vi "ObserverPattern_Demo_Main.vi"() -> ()   [LabVIEW 2010]
uses:
  WeatherData.ctl
  ForecastConditionDisplay_class/ForecastConditionDisplay.lvclass
  CurrentConditionDisplay_class/CurrentConditionDisplay.lvclass
  WeatherStation_class/WeatherStation.lvclass
panel:
  out "No.OfObservers":i32
  in  "Forecast.Subscribe?":bool caption="Subscribe?"
  in  "Subscribe?":bool
  out "Forecast message":string
  out "Forecast Temperature F":dbl(slide) scale=0.0..160.0
  out "Forecast":string
  out "Humid %":dbl(knob) scale=0.0..100.0
  out "CurrentTemperature C":dbl(slide) scale=0.0..60.0
  in  "stop":bool
  in  "error in (no error)":errorcluster
  in  "WeatherData-Acquired":T1
  # "CURRENT CONDITION"
  # "FORECAST"
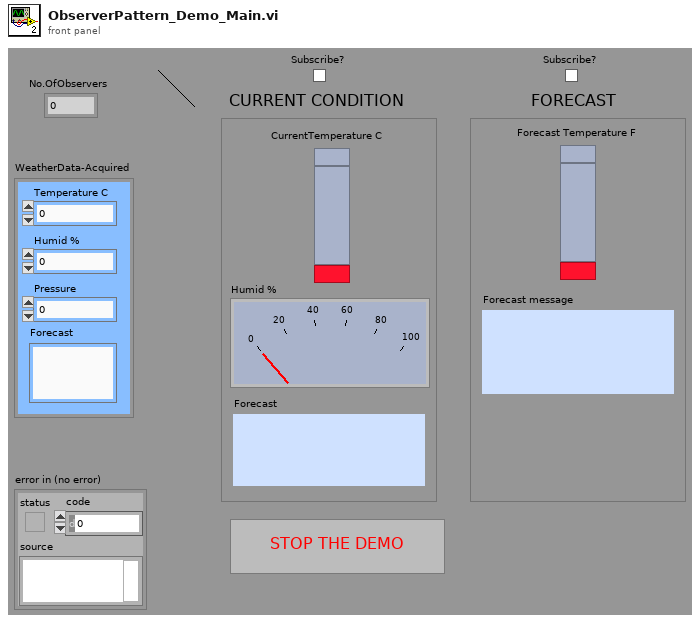
[diagram p1: front panel]
types:
  T1 = typedef "WeatherData.ctl" = cluster{"Temperature C":dbl, "Humid %":dbl, "Pressure":dbl, "Forecast":string}
  T2 = cluster{"No.OfObservers":i32, "CurrentDisplaySubscribe?":bool, "ForecastDisplaySubscribe?":bool, "WSRef":refnum<class "WeatherStation.lvclass">, "ForecastDisplayRef":refnum<class "ForecastConditionDisplay.lvclass">, "CurrentDisplayRef":refnum<class "CurrentConditionDisplay.lvclass">}
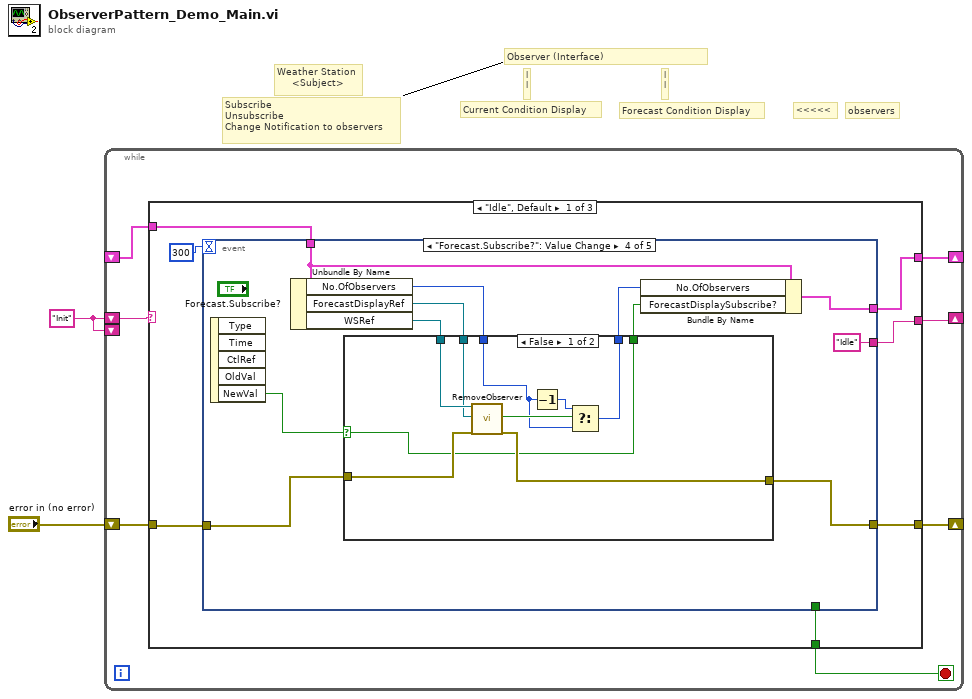
[diagram p0: block diagram]
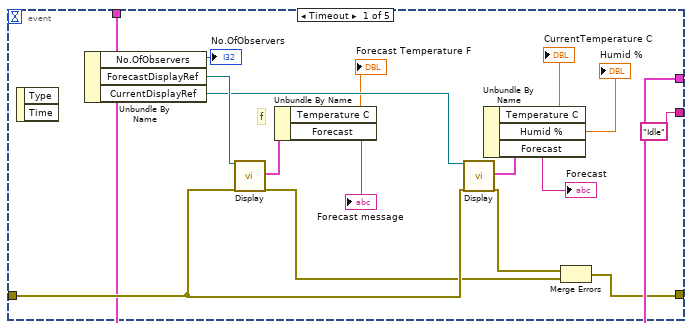
[diagram p2: hidden frame]
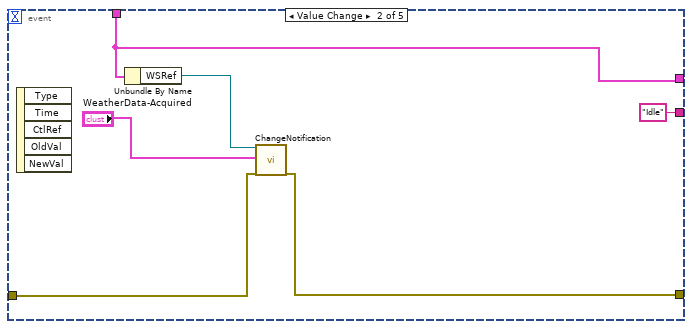
[diagram p3: hidden frame]
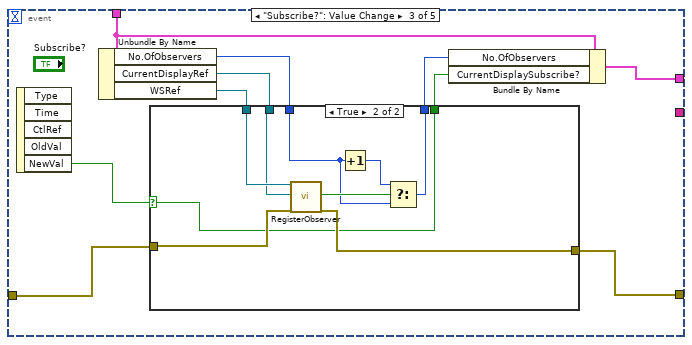
[diagram p4: hidden frame]
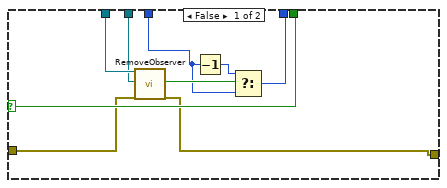
[diagram p5: hidden frame]
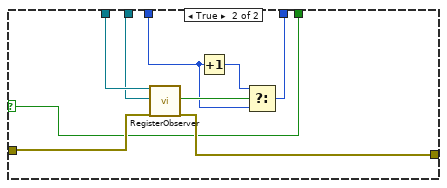
[diagram p6: hidden frame]
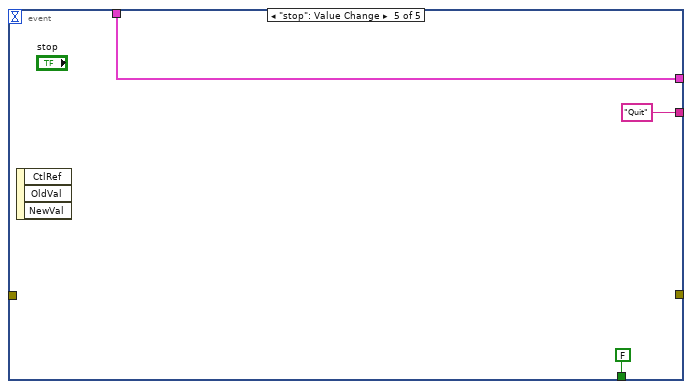
[diagram p7: hidden frame]
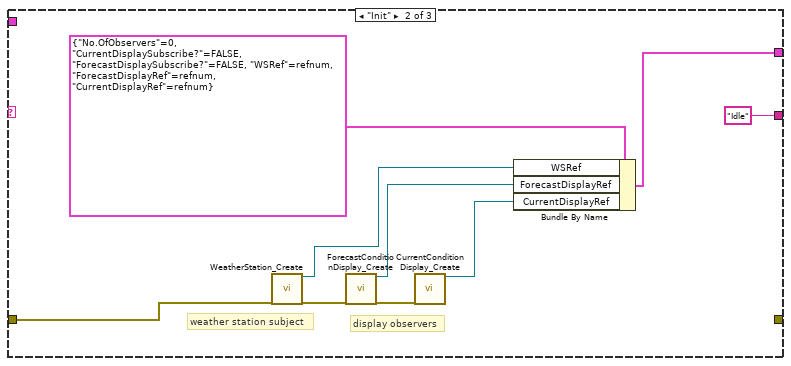
[diagram p8: hidden frame]
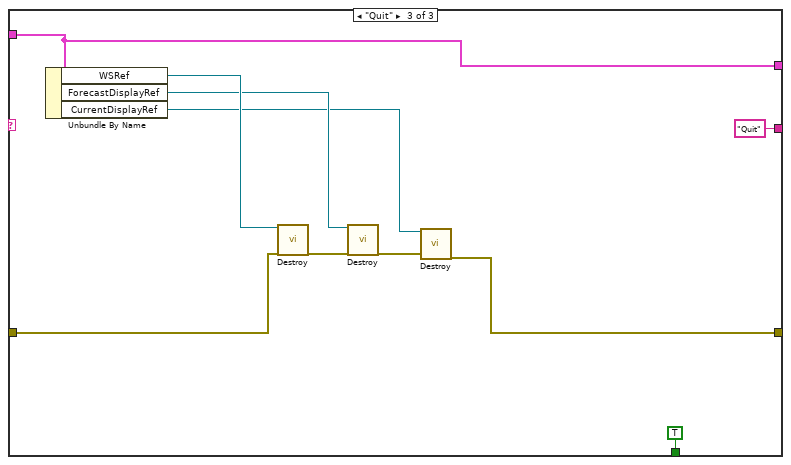
[diagram p9: hidden frame]
diagram:
  w2 = "Init"
  # "<<<<<"
  # "observers"
  # "Subscribe\nUnsubscribe\nChange Notification to observers"
  # "l\nl"
  # "Forecast Condition Display"
  # "l\nl"
  # "Current Condition Display"
  # "Observer (Interface)"
  # "Weather Station\n     <Subject>"
  n1 = while {
    shift-right: [w6] -> _
    shift-left: w2 -> [w9]
    shift-left: w2 -> [_]
    shift-right: [w3] -> _
    shift-left: "error in (no error)" -> [w8]
    shift-right: [w7] -> _
    shift-left: _ -> [w5]
    stop <- w4 stop-if-true
    n2 = case shown="\"Idle\", Default" w9 {
      tunnel: w8 -> [w11 w107 w109]
      tunnel: [w13 w100 w115] -> w7
      tunnel: [w12 "Idle" "Quit"] -> w6
      tunnel: w5 -> [w15 _ w115]
      tunnel: [w14 _ TRUE] -> w4
      tunnel: [w10 _ w108] -> w3
      frame "Idle", Default {
        n3 = event shown="[3] \"Forecast.Subscribe?\": Value Change" {
          selector: _ -> [_ _ _ _ _]
          dyn-events: _ -> [_ _ _ _ _]
          timeout: 300 -> [_ _ _ _ _]
          tunnel: w15 -> [w22 w35 w42 w71 w97]
          tunnel: [_ _ _ _ FALSE] -> w14
          tunnel: [w22 w35 w39 w68 w97] -> w13
          tunnel: ["Idle" "Idle" _ "Idle" "Quit"] -> w12
          tunnel: w11 -> [w29 w37 w47 w76 _]
          tunnel: [w17 w36 w43 w72 _] -> w10
          event Timeout {
            # "f"
            n4 = event-data() -> ()  [unwired: 1 in, 2 out]
            n5 = Unbundle By Name(w22) -> ("No.OfObservers"=→"No.OfObservers":i32, "ForecastDisplayRef"=w31:refnum<class "ForecastConditionDisplay.lvclass">, "CurrentDisplayRef"=w30:refnum<class "CurrentConditionDisplay.lvclass">)
            n6 = call-dynamic "Display.vi"("reference in"=w31, "error in (no error)"=w29) -> ("WeatherData"=w28:T1, "error out"=w19:errorcluster)  [unwired: 15 in, 1 out]
            n7 = Unbundle By Name(w28) -> ("Temperature C"=→"Forecast Temperature F":dbl, "Forecast"=→"Forecast message":string)
            n8 = call-dynamic "Display.vi"("reference in"=w30, "error in (no error)"=w29) -> ("WeatherData"=w25:T1, "error out"=w18:errorcluster)  [unwired: 15 in, 1 out]
            n9 = Unbundle By Name(w25) -> ("Temperature C"=→"CurrentTemperature C":dbl, "Humid %"=→"Humid %":dbl, "Forecast"=→"Forecast":string)
            n10 = Merge Errors(w18, w19) -> (w17:errorcluster)
          }
          event Value Change {
            n11 = event-data() -> ()  [unwired: 1 in, 5 out]
            n12 = Unbundle By Name(w35) -> ("WSRef"=w38:refnum<class "WeatherStation.lvclass">)
            n13 = call-dynamic "ChangeNotification.vi"("reference in"=w38, "WeatherData"="WeatherData-Acquired", "error in (no error)"=w37) -> ("error out"=w36:errorcluster)  [unwired: 15 in, 1 out]
          }
          event "Subscribe?": Value Change {
            n14 = event-data() -> ("NewVal"=w48:bool)  [unwired: 1 in, 4 out]
            n15 = Unbundle By Name(w42) -> ("No.OfObservers"=w46:i32, "CurrentDisplayRef"=w45:refnum<class "CurrentConditionDisplay.lvclass">, "WSRef"=w44:refnum<class "WeatherStation.lvclass">)
            n16 = case shown="True" w48 {
              selector: w48 -> [w57 w58]
              tunnel: w47 -> [w54 w64]
              tunnel: w46 -> [w50 w61]
              tunnel: w45 -> [w55 w65]
              tunnel: w44 -> [w56 w66]
              tunnel: [w53 w60] -> w43
              tunnel: [w49 w59] -> w41
              tunnel: [w57 w58] -> w40
              frame False {
                n17 = call-dynamic "RemoveObserver.vi"("reference in"=w56, "Observer"=w55, "error in (no error)"=w54) -> ("Removed?"=w52:bool, "error out"=w53:errorcluster)  [unwired: 14 in, 1 out]
                n18 = Decrement(x=w50) -> (x-1=w51:i32)
                n19 = Select(t=w51, s=w52, f=w50) -> (s? t:f=w49:i32)
              }
              frame True {
                n20 = call-dynamic "RegisterObserver.vi"("reference in"=w66, "Observer"=w65, "error in (no error)"=w64) -> ("Added?"=w63:bool, "error out"=w60:errorcluster)  [unwired: 14 in, 1 out]
                n21 = Increment(x=w61) -> (x+1=w62:i32)
                n22 = Select(t=w62, s=w63, f=w61) -> (s? t:f=w59:i32)
              }
            }
            n23 = Bundle By Name(cluster=w42, "No.OfObservers"=w41, "CurrentDisplaySubscribe?"=w40) -> (w39:T2)
          }
          event "Forecast.Subscribe?": Value Change {
            n24 = event-data() -> ("NewVal"=w77:bool)  [unwired: 1 in, 4 out]
            n25 = Unbundle By Name(w71) -> ("No.OfObservers"=w75:i32, "ForecastDisplayRef"=w74:refnum<class "ForecastConditionDisplay.lvclass">, "WSRef"=w73:refnum<class "WeatherStation.lvclass">)
            n26 = case shown="False" w77 {
              selector: w77 -> [w78 w87]
              tunnel: w76 -> [w82 w93]
              tunnel: w75 -> [w80 w90]
              tunnel: w74 -> [w83 w94]
              tunnel: w73 -> [w84 w95]
              tunnel: [w81 w89] -> w72
              tunnel: [w79 w88] -> w70
              tunnel: [w78 w87] -> w69
              frame False {
                n27 = call-dynamic "RemoveObserver.vi"("reference in"=w84, "Observer"=w83, "error in (no error)"=w82) -> ("Removed?"=w86:bool, "error out"=w81:errorcluster)  [unwired: 14 in, 1 out]
                n28 = Decrement(x=w80) -> (x-1=w85:i32)
                n29 = Select(t=w85, s=w86, f=w80) -> (s? t:f=w79:i32)
              }
              frame True {
                n30 = call-dynamic "RegisterObserver.vi"("reference in"=w95, "Observer"=w94, "error in (no error)"=w93) -> ("Added?"=w92:bool, "error out"=w89:errorcluster)  [unwired: 14 in, 1 out]
                n31 = Increment(x=w90) -> (x+1=w91:i32)
                n32 = Select(t=w91, s=w92, f=w90) -> (s? t:f=w88:i32)
              }
            }
            n33 = Bundle By Name(cluster=w71, "No.OfObservers"=w70, "ForecastDisplaySubscribe?"=w69) -> (w68:T2)
          }
          event "stop": Value Change {
            n34 = event-data() -> ()  [unwired: 1 in, 3 out]
          }
        }
      }
      frame "Init" {
        # "weather station subject"
        # "display observers"
        n35 = call "WeatherStation_Create.vi"("error in (no error)"=w107) -> ("reference out"=w103:refnum<class "WeatherStation.lvclass">, "error out"=w106:errorcluster)  [unwired: 17 in]
        n36 = call "ForecastConditionDisplay_Create.vi"("error in (no error)"=w106) -> ("reference out"=w102:refnum<class "ForecastConditionDisplay.lvclass">, "error out"=w105:errorcluster)  [unwired: 17 in]
        n37 = call "CurrentConditionDisplay_Create.vi"("error in (no error)"=w105) -> ("reference out"=w101:refnum<class "CurrentConditionDisplay.lvclass">)  [unwired: 17 in, 1 out]
        n38 = Bundle By Name(cluster=T2 {"No.OfObservers"=0, "CurrentDisplaySubscribe?"=FALSE, "ForecastDisplaySubscribe?"=FALSE, "WSRef"=refnum, "ForecastDisplayRef"=refnum, "CurrentDisplayRef"=refnum}, "WSRef"=w103, "ForecastDisplayRef"=w102, "CurrentDisplayRef"=w101) -> (w100:T2)
      }
      frame "Quit" {
        n39 = Unbundle By Name(w115) -> ("WSRef"=w114:refnum<class "WeatherStation.lvclass">, "ForecastDisplayRef"=w113:refnum<class "ForecastConditionDisplay.lvclass">, "CurrentDisplayRef"=w112:refnum<class "CurrentConditionDisplay.lvclass">)
        n40 = call-dynamic "Destroy.vi"("reference in"=w114, "error in (no error)"=w109) -> ("error out"=w111:errorcluster)  [unwired: 16 in, 1 out]
        n41 = call-dynamic "Destroy.vi"("reference in"=w113, "error in (no error)"=w111) -> ("error out"=w110:errorcluster)  [unwired: 16 in, 1 out]
        n42 = call-dynamic "Destroy.vi"("reference in"=w112, "error in (no error)"=w110) -> ("error out"=w108:errorcluster)  [unwired: 16 in, 1 out]
      }
    }
  }
